vi "_Initialize.vi"(11 "Force Simulation (F)":bool) -> (0 "error":errorcluster, 1 "InstrState":T2, 3 "FPGA VI Reference Out":T1, 5 "FPGA Version":u32)   [LabVIEW 2015]
uses:
  Type/_RT Instrument State.ctl
  Type/FPGA Typedef.ctl
  _RT Global.vi
  <vilib>/FPGAPlugInAG/sbRIO-9607/niLvFpga_Close_sbRIO-9607.vi
  <vilib>/FPGAPlugInAG/sbRIO-9607/niLvFpga_Open_sbRIO-9607.vi
  <vilib>/Utility/error.llb/Error Cluster From Error Code.vi
  <vilib>/rvi/interface/common/niFpgaWaitOnOcc.vi
  <vilib>/FPGAPlugInAG/sbRIO-9607/niLvFpga_Run_sbRIO-9607.vi
  <vilib>/rvi/errors/niLvFpgaAdjustHostInterfaceError.vi
  <vilib>/Utility/config.llb/Read Key (Boolean).vi
  <vilib>/Utility/config.llb/Read Key (String).vi
  <vilib>/rvi/interface/nirviCloseFPGA/nirviCloseFPGA.xnode
  FPGA Bitfiles/FPGA9607.lvbitx
  <vilib>/rvi/interface/nirviOpenFPGA/nirviOpenFPGA.xnode
  <vilib>/rvi/interface/nirviMethod/nirviMethod.xnode
  <vilib>/rvi/interface/nirviReadWriteControl/nirviReadWriteControl.xnode
  <vilib>/rvi/errors/niLvFpgaMergeErrorWithErrorCode.vi
  <vilib>/Utility/config.llb/NI_LVConfig.lvlib
  <vilib>/FPGAPlugInAG/sbRIO-9607/niLvFpga_StopFifo_sbRIO-9607.vi
  <vilib>/FPGAPlugInAG/sbRIO-9607/niLvFpga_ConfigureFifo_sbRIO-9607.vi
  <vilib>/FPGAPlugInAG/sbRIO-9607/niLvFpga_StartFifo_sbRIO-9607.vi
  NiFpgaLv.dll
panel:
  out "FilePath":path
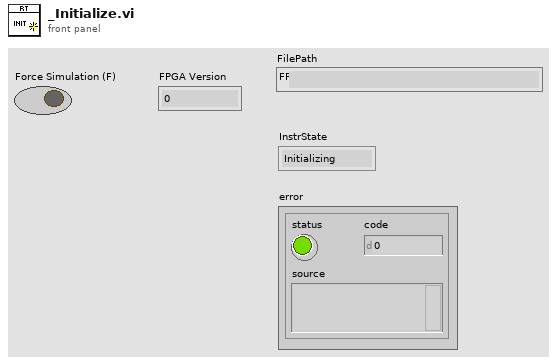
[diagram p1: front panel]
types:
  T1 = typedef "FPGA Typedef.ctl" = refnum<k20>
  T2 = typedef "_RT Instrument State.ctl" = enum16{"Initializing", "Mass Spectrometer is Off", "Starting Up", "Turning Power Off", "Going to Standby", "Roughing Pump Ready", "Turning Turbo Off", "Turbo Startup", "Turbopump Ready", "Checking Vacuum", "Going to Ready", "Ready", "Running", "Source Standby", "Lost Communication", "Shutting Down", "Fault", "24V Standby", "Go to 24V Standby", "Turbopump Ready-Waiting"}
  T3 = enum16{"open", "replace", "create", "open or create", "replace or create", "replace or create with confirmation"}
  T4 = typedef "_RT Instrument 2.ctl" = cluster{"Table":T5[], "Instrument":string[]}
  T5 = typedef "_RT Configuration 2.ctl" = cluster{"Name":string, "Ch#":u8, "Min":dbl, "Max":dbl, "Def+":dbl, "Def-":dbl, "Offset":dbl, "Slope":dbl, "Type":u8, "Description":string, "SettleT":dbl}
  T6 = typedef "Semaphore RefNum" = refnum<k1>
  T7 = typedef "NI_LVConfig.lvlib/Config Data RefNum.ctl" = refnum<k1>
  T8 = typedef "_RT Startup Options.ctl" = cluster{"Door":bool, "Curtain":bool, "Pressure":bool, "Turbo":bool, "SysPoll":bool, "GasFlag":bool, "SourceExhaust":bool}
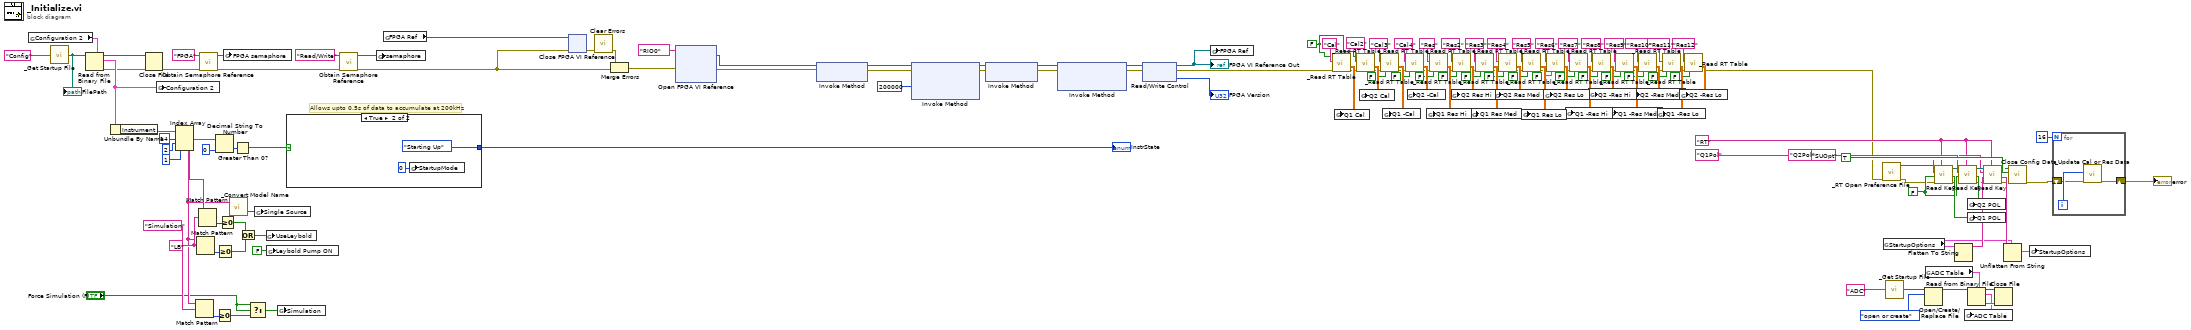
[diagram p0: block diagram]
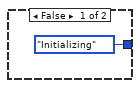
[diagram p2: hidden frame]
diagram:
  w31 = FALSE ("Connected?")
  w26 = "RT" ("section")
  (unwired) FALSE ("Simulator")
  w66 = FALSE ("Simulator")
  w146 = "LB" ("regular expression")
  # "Allows upto 0.5s of data to accumulate at 200kHz"
  n1 = global read "_RT Global.vi" "Configuration 2"() -> (w120:T4)
  n2 = call "_Get Startup File.vi"("FileName"="Config" ("key")) -> ("FilePath"=w139:path)
  "FilePath" <- w139
  n3 = Read from Binary File(5:w120, 11:w139) -> (0:w121:errorcluster, 2:w123:T4, 3:w122:refnum<file>)  [unwired: 1 in, 4 out]
  n4 = Unbundle By Name(w123) -> ("Instrument"=w124:string[])
  n5 = Close File(refnum=w122, error in=w121) -> (error out=w149:errorcluster)  [unwired: 1 out]
  n6 = global write "_RT Global.vi" "Configuration 2"(w123) -> ()
  n7 = Index Array(array=w124, index #1=14 ("index"), index #2=2 ("index"), index #3=1 ("index")) -> (element #1=w127:string, element #2=w142:string, element #3=w145:string)
  n8 = Match Pattern(string=w142, regular expression="Simulation") -> (offset past match=w136:i32)  [unwired: 4 out]
  n9 = Match Pattern(string=w142, regular expression=w146) -> (offset past match=w141:i32)  [unwired: 4 out]
  n10 = Match Pattern(string=w145, regular expression=w146) -> (offset past match=w144:i32)  [unwired: 4 out]
  n11 = call <vilib>:"Obtain Semaphore Reference.vi"("error in (no error)"=w149, "name (unnamed)"="FPGA") -> ("error out"=w132:errorcluster, "semaphore"=w134:T6)  [unwired: 1 in, 3 out]
  n12 = Decimal String To Number(string=w127, default (0L)=0 ("default (0 I32)")) -> (number=w128:i32)  [unwired: 2 out]
  n13 = Greater Or Equal To 0?(x=w136) -> (x >= 0?=w114:bool)
  n14 = Greater Or Equal To 0?(x=w141) -> (x >= 0?=w147:bool)
  n15 = Greater Or Equal To 0?(x=w144) -> (x >= 0?=w148:bool)
  n16 = global write "_RT Global.vi" "FPGA semaphore"(w134) -> ()
  n17 = call "_Convert Model Name.vi"("Model"=w142) -> ("SingleSource"=w138:bool)  [unwired: 1 in, 1 out]
  n18 = Greater Than 0?(x=w128) -> (x > 0?=w129:bool)
  n19 = Or(x=w148, y=w147) -> (x .or. y?=w2:bool)
  n20 = Select(t="Force Simulation (F)", s="Force Simulation (F)", f=w114) -> (s? t:f=w115:bool)
  n21 = global write "_RT Global.vi" "Single Source"(w138) -> ()
  n22 = global write "_RT Global.vi" "UseLeybold"(w2) -> ()
  n23 = global write "_RT Global.vi" "Leybold Pump ON"(FALSE ("Leybold Pump ON")) -> ()
  n24 = global write "_RT Global.vi" "Simulation"(w115) -> ()
  n25 = case shown="True" w129 {
    tunnel: [_RT_Instrument_State."Initializing" ("InstrState") _RT_Instrument_State."Starting Up" ("InstrState")] -> w119
    frame False {
    }
    frame True {
      n26 = global write "_RT Global.vi" "StartupMode"(u8 0 ("StartupMode")) -> ()
    }
  }
  "InstrState" <- w119
  n27 = call <vilib>:"Obtain Semaphore Reference.vi"("error in (no error)"=w132, "name (unnamed)"="Read/Write") -> ("error out"=w3:errorcluster, "semaphore"=w130:T6)  [unwired: 1 in, 3 out]
  n28 = global write "_RT Global.vi" "semaphore"(w130) -> ()
  n29 = global read "_RT Global.vi" "FPGA Ref"() -> (w109:T1)
  n30 = xnode "Close FPGA VI Reference"("FPGA VI Reference In"=w109, "error in"=w3) -> ("error out"=w112:errorcluster)
  n31 = call <vilib>:"Clear Errors.vi"("error in (no error)"=w112) -> ("error out"=w111:errorcluster)  [unwired: 5 in, 1 out]
  n32 = Merge Errors(w111, w3) -> (w110:errorcluster)
  n33 = xnode "Open FPGA VI Reference"("error in"=w110, "resource name"=tag "RIO0") -> ("FPGA VI Reference Out"=w7:T1, "error out"=w8:errorcluster)
  n34 = xnode "Invoke Method"("FPGA VI Reference In"=w7, "error in"=w8) -> ("FPGA VI Reference Out"=w106:T1, "error out"=w107:errorcluster)
  n35 = xnode "Invoke Method"("FPGA VI Reference In"=w106, "error in"=w107, "Requested Depth"=u32 200000 ("Depth")) -> ("FPGA VI Reference Out"=w117:T1, "error out"=w116:errorcluster)  [unwired: 1 out]
  n36 = xnode "Invoke Method"("FPGA VI Reference In"=w117, "error in"=w116) -> ("FPGA VI Reference Out"=w103:T1, "error out"=w104:errorcluster)
  n37 = xnode "Invoke Method"("FPGA VI Reference In"=w103, "error in"=w104) -> ("FPGA VI Reference Out"=w101:T1, "error out"=w102:errorcluster)  [unwired: 1 in]
  n38 = xnode "Read/Write Control"("FPGA VI Reference In"=w101, "error in"=w102) -> ("FPGA VI Reference Out"=w108:T1, "error out"=w99:errorcluster, "Version"=→"FPGA Version":u32)
  "FPGA VI Reference Out" <- w108
  n39 = global write "_RT Global.vi" "FPGA Ref"(w108) -> ()
  n40 = call "_Read RT Table.vi"("error in (no error)"=w99, "key"="Cal", "Simulator"=w66) -> ("error out"=w52:errorcluster, "Table"=w67:dbl[][])  [unwired: 1 in, 2 out]
  n41 = global write "_RT Global.vi" "Q1 Cal"(w67) -> ()
  n42 = call "_Read RT Table.vi"("error in (no error)"=w52, "key"="Cal2", "Simulator"=w66) -> ("error out"=w51:errorcluster, "Table"=w68:dbl[][])  [unwired: 1 in, 2 out]
  n43 = global write "_RT Global.vi" "Q2 Cal"(w68) -> ()
  n44 = call "_Read RT Table.vi"("error in (no error)"=w51, "key"="Cal3", "Simulator"=FALSE) -> ("error out"=w50:errorcluster, "Table"=w69:dbl[][])  [unwired: 1 in, 2 out]
  n45 = global write "_RT Global.vi" "Q1 -Cal"(w69) -> ()
  n46 = call "_Read RT Table.vi"("error in (no error)"=w50, "key"="Cal4", "Simulator"=FALSE) -> ("error out"=w49:errorcluster, "Table"=w70:dbl[][])  [unwired: 1 in, 2 out]
  n47 = global write "_RT Global.vi" "Q2 -Cal"(w70) -> ()
  n48 = call "_Read RT Table.vi"("error in (no error)"=w49, "key"="Res", "Simulator"=FALSE) -> ("error out"=w48:errorcluster, "Table"=w71:dbl[][])  [unwired: 1 in, 2 out]
  n49 = global write "_RT Global.vi" "Q1 Res Hi"(w71) -> ()
  n50 = call "_Read RT Table.vi"("error in (no error)"=w48, "key"="Res2", "Simulator"=FALSE) -> ("error out"=w47:errorcluster, "Table"=w72:dbl[][])  [unwired: 1 in, 2 out]
  n51 = global write "_RT Global.vi" "Q2 Res Hi"(w72) -> ()
  n52 = call "_Read RT Table.vi"("error in (no error)"=w47, "key"="Res3", "Simulator"=FALSE) -> ("error out"=w46:errorcluster, "Table"=w73:dbl[][])  [unwired: 1 in, 2 out]
  n53 = global write "_RT Global.vi" "Q1 Res Med"(w73) -> ()
  n54 = call "_Read RT Table.vi"("error in (no error)"=w46, "key"="Res4", "Simulator"=FALSE) -> ("error out"=w45:errorcluster, "Table"=w74:dbl[][])  [unwired: 1 in, 2 out]
  n55 = global write "_RT Global.vi" "Q2 Res Med"(w74) -> ()
  n56 = call "_Read RT Table.vi"("error in (no error)"=w45, "key"="Res5", "Simulator"=FALSE) -> ("error out"=w44:errorcluster, "Table"=w75:dbl[][])  [unwired: 1 in, 2 out]
  n57 = global write "_RT Global.vi" "Q1 Res Lo"(w75) -> ()
  n58 = call "_Read RT Table.vi"("error in (no error)"=w44, "key"="Res6") -> ("error out"=w43:errorcluster, "Table"=w76:dbl[][])  [unwired: 2 in, 2 out]
  n59 = global write "_RT Global.vi" "Q2 Res Lo"(w76) -> ()
  n60 = call "_Read RT Table.vi"("error in (no error)"=w43, "key"="Res7", "Simulator"=FALSE) -> ("error out"=w42:errorcluster, "Table"=w77:dbl[][])  [unwired: 1 in, 2 out]
  n61 = global write "_RT Global.vi" "Q1 -Res Hi"(w77) -> ()
  n62 = call "_Read RT Table.vi"("error in (no error)"=w42, "key"="Res8", "Simulator"=FALSE) -> ("error out"=w41:errorcluster, "Table"=w78:dbl[][])  [unwired: 1 in, 2 out]
  n63 = global write "_RT Global.vi" "Q2 -Res Hi"(w78) -> ()
  n64 = call "_Read RT Table.vi"("error in (no error)"=w41, "key"="Res9", "Simulator"=FALSE) -> ("error out"=w40:errorcluster, "Table"=w79:dbl[][])  [unwired: 1 in, 2 out]
  n65 = global write "_RT Global.vi" "Q1 -Res Med"(w79) -> ()
  n66 = call "_Read RT Table.vi"("error in (no error)"=w40, "key"="Res10", "Simulator"=FALSE) -> ("error out"=w39:errorcluster, "Table"=w80:dbl[][])  [unwired: 1 in, 2 out]
  n67 = global write "_RT Global.vi" "Q2 -Res Med"(w80) -> ()
  n68 = call "_Read RT Table.vi"("error in (no error)"=w39, "key"="Res11", "Simulator"=FALSE) -> ("error out"=w38:errorcluster, "Table"=w81:dbl[][])  [unwired: 1 in, 2 out]
  n69 = global write "_RT Global.vi" "Q1 -Res Lo"(w81) -> ()
  n70 = call "_Read RT Table.vi"("error in (no error)"=w38, "key"="Res12", "Simulator"=FALSE) -> ("error out"=w6:errorcluster, "Table"=w82:dbl[][])  [unwired: 1 in, 2 out]
  n71 = global write "_RT Global.vi" "Q2 -Res Lo"(w82) -> ()
  n72 = call "_RT Open Preference File.vi"("error In"=w6) -> ("error"=w12:errorcluster, "refnum"=w30:T7)  [unwired: 5 out]
  n73 = global read "_RT Global.vi" "StartupOptions"() -> (w21:T8)
  n74 = call "_Get Startup File.vi"("FileName"="ADC" ("key")) -> ("FilePath"=w14:path)
  n75 = Open/Create/Replace File(file path (use dialog)=w14, operation (0:open)=T3."open or create") -> (refnum out=w13:refnum<file>)  [unwired: 4 in, 2 out]
  n76 = global read "_RT Global.vi" "ADC Table"() -> (w17:T5[])
  n77 = call-poly <vilib>:"Read Key.vi"("section"=w26, "error in (no error)"=w12, "default value"=w31, "key"="Q1Pol", "refnum"=w30) -> ("error out"=w11:errorcluster, "value"=w32:bool, "refnum out"=w33:T7)  [unwired: 4 out]
  n78 = Flatten To String(anything=w21) -> (data string=w24:string)  [unwired: 1 in, 4 out]
  n79 = call-poly <vilib>:"Read Key.vi"("section"=w26, "error in (no error)"=w11, "default value"=w31, "key"="Q2Pol", "refnum"=w33) -> ("error out"=w10:errorcluster, "value"=w29:bool, "refnum out"=w28:T7)  [unwired: 4 out]
  n80 = global write "_RT Global.vi" "Q2 POL"(w29) -> ()
  n81 = global write "_RT Global.vi" "Q1 POL"(w32) -> ()
  n82 = Read from Binary File(5:w17, 11:w13) -> (0:w19:errorcluster, 2:w18:T5[], 3:w20:refnum<file>)  [unwired: 1 in, 4 out]
  n83 = global write "_RT Global.vi" "ADC Table"(w18) -> ()
  n84 = call-poly <vilib>:"Read Key.vi"("section"=w26, "error in (no error)"=w10, "default value"=w24, "key"="SUOpt", "refnum"=w28) -> ("error out"=w9:errorcluster, "value"=w23:string, "refnum out"=w25:T7)  [unwired: 1 in, 3 out]
  n85 = Close File(refnum=w20, error in=w19) -> ()  [unwired: 2 out]
  n86 = Unflatten From String(type=w21, binary string=w23) -> (value=w22:T8)  [unwired: 1 in, 4 out]
  n87 = call <vilib>:"Close Config Data.vi"("error in (no error)"=w9, "write file if changed (T)"=TRUE ("write configuration file? (T)"), "refnum"=w25) -> ("error out"=w5:errorcluster)  [unwired: 8 out]
  n88 = global write "_RT Global.vi" "StartupOptions"(w22) -> ()
  n89 = for {
    N: 16 -> [_]
    shift-right: [w154] -> w4
    shift-left: w5 -> [w153]
    i -> [w155]
    n90 = call "_Update Cal or Res Data.vi"("error in (no error)"=w153, "Table Type"=w155) -> ("error out"=w154:errorcluster)  [unwired: 1 in, 4 out]
  }
  "error" <- w4
